vi "SV Continuous Swept-Sine THD+N.vi"(0 "scaled signals [EU]":waveform(dbl)[](array[waveform]), 1 "desired units":T3, 2 "reset? (F)":bool, 7 "harmonic range":cluster{"start order":dbl, "stop order":dbl}={"start order"=-1.0, "stop order"=-1.0} {"stop order" format="%.2f"; "start order" format="%.2f"}, 9 "advanced span [order]":dbl=1.0 format="%0.2f", 11 "error in (no error)":errorcluster, 12 "buffer settings":T2 {"buffer mode" items=["Infinite length", "Last block data", "Custom"]}, 13 "zero delay? (F)":bool) -> (3 "unit labels":T1(array[cluster]), 4 "scaled signals out [EU]":waveform(dbl)[](array[waveform]), 6 "THD+N":cluster{"frequency":dbl[], "amplitude":dbl[]}[](array[cluster]) {"amplitude" format="%.2f"; "frequency" format="%.2f"}, 8 "SINAD":cluster{"frequency":dbl[], "amplitude":dbl[]}[](array[cluster]) {"amplitude" format="%.2f"; "frequency" format="%.2f"}, 15 "error out":errorcluster)   [LabVIEW 2017, in "SoundVib_ContSweptSine.lvlib"]
doc: "Computes the total harmonic distortion plus noise (THD+N) and signal in noise and distortion (SINAD) of the input signals by performing a continuous swept-sine measurement."
uses:
  <vilib>/addons/Sound and Vibration/svt_Continuous Swept Sine/SoundVib_ContSweptSine.lvlib
  <vilib>/addons/_NISVFA/_Shared subVIs/Controls/sv_Buffer XY Settings.ctl
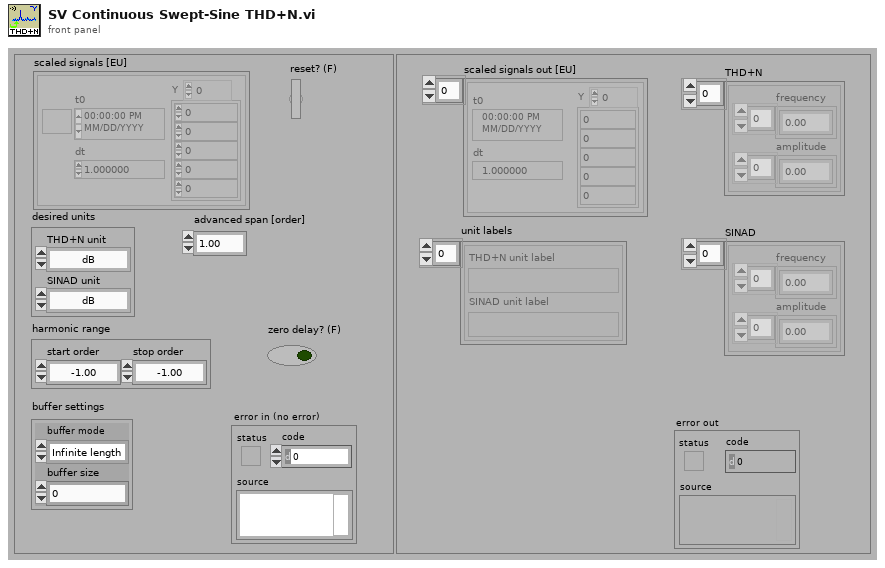
[diagram p1: front panel]
types:
  T1 = cluster{"THD+N unit label":string, "SINAD unit label":string}[]
  T2 = typedef "sv_Buffer XY Settings.ctl" = cluster{"buffer mode":u16, "buffer size":dbl}
  T3 = cluster{"THD+N unit":enum16{"dB", "linear ratio", "%"}, "SINAD unit":enum16{"dB", "linear ratio", "%"}}
  T4 = typedef "svc_Resampled Channel Info.ctl" = cluster{"channel name":string, "description":string, " channel info":T5}
  T5 = typedef "svc_Channel Info.ctl" = cluster{"sensor sensitivity":dbl, "engineering units":T6, "dB reference":dbl, "custom label":string, "weighting filter":T7, "pregain":dbl}
  T6 = typedef "svc_Engineering Units Text Ring.ctl" = u16
  T7 = typedef "svc_Weighting Filter Text Ring.ctl" = u16
  T8 = typedef "OAT Position Info.ctl" = cluster{"positions [s]":dbl[], "samples/rev":dbl}
  T9 = cluster{"THD+N unit":string, "SINAD unit":string}[]
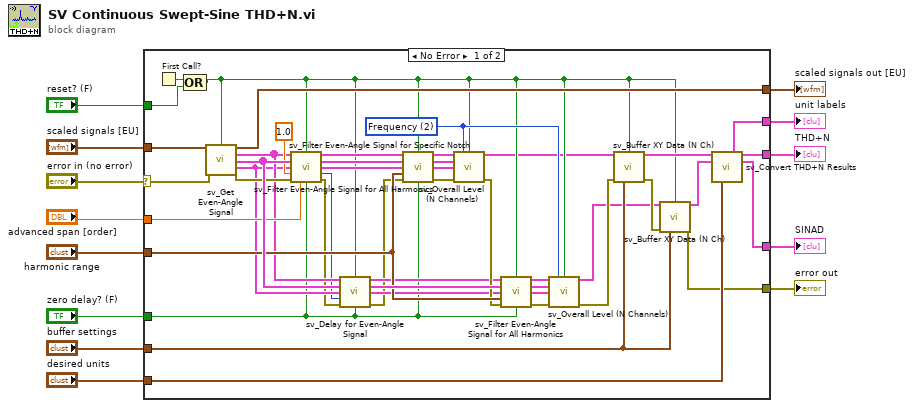
[diagram p0: block diagram]
diagram:
  n1 = case shown="No Error" "error in (no error)" {
    selector: "error in (no error)" -> [w54 w56]
    tunnel: [w35 w56] -> w12
    tunnel: "scaled signals [EU]" -> [w53 w55]
    tunnel: [w45 w55] -> w10
    tunnel: "desired units" -> [w36 _]
    tunnel: "harmonic range" -> [w29 _]
    tunnel: [w39 _] -> w7
    tunnel: [w38 _] -> w2
    tunnel: "buffer settings" -> [w44 _]
    tunnel: "zero delay? (F)" -> [w17 _]
    tunnel: "reset? (F)" -> [w46 _]
    tunnel: [w37 _] -> w3
    tunnel: "advanced span [order]" -> [w30 _]
    frame No Error {
      w50 = u16 2 items=["Time", "Revolution", "Frequency"] ("x-axis selection")
      n2 = First Call?() -> (First Call?: T/F=w47:bool)
      n3 = Compound Arithmetic op=OR(w47, w46) -> (w20:bool)
      n4 = call <vilib>:"sv_Get Even-Angle Signal.vi"("data to process"=w53, "reset?"=w20, "error in (no error)"=w54) -> ("data to process out"=w45:waveform(dbl)[], "even-angle signals"=w24:cluster{"r0":dbl, "dr":dbl, "Y":dbl[]}[], "even-angle channel info"=w52:T4[], "even-angle position info"=w22:T8, "error out"=w31:errorcluster)  [unwired: 7 in, 1 out]
      n5 = call <vilib>:"sv_Filter Even-Angle Signal for Specific Notch.vi"("even-angle signals"=w24, "reset?"=w20, "even-angle position info"=w22, "notch harmonic"=1.0, "error in (no error)"=w31, "bandwidth [order]"=w30, "zero delay? (F)"=w17) -> ("even-angle signals out"=w34:cluster{"r0":dbl, "dr":dbl, "Y":dbl[]}[], "even-angle position info out"=w33:T8, "delay [samples]"=w19:i32, "error out"=w18:errorcluster)  [unwired: 5 in]
      n6 = call <vilib>:"sv_Delay for Even-Angle Signal.vi"("even-angle signals"=w24, "reset?"=w20, "even-angle position info"=w22, "delay [samples]"=w19, "error in (no error)"=w18, "zero delay? (F)"=w17) -> ("even-angle signals out"=w23:cluster{"r0":dbl, "dr":dbl, "Y":dbl[]}[], "even-angle position info out"=w21:T8, "error out"=w16:errorcluster)  [unwired: 7 in]
      n7 = call <vilib>:"sv_Filter Even-Angle Signal for All Harmonics.vi"("even-angle signals"=w34, "reset?"=w20, "even-angle position info"=w33, "harmonic range"=w29, "error in (no error)"=w16, "zero delay? (F)"=w17) -> ("even-angle signals out"=w49:cluster{"r0":dbl, "dr":dbl, "Y":dbl[]}[], "even-angle position info out"=w48:T8, "error out"=w51:errorcluster)  [unwired: 7 in]
      n8 = call <vilib>:"sv_Overall Level (N Channels).vi"("even-angle signals"=w49, "x-axis selection"=w50, "reset? (F)"=w20, "even-angle channel info"=w52, "even-angle position info"=w48, "error in (no error)"=w51) -> ("overall levels"=w15:cluster{"time/rev/rpm":dbl[], "level":dbl[]}[], "error out"=w26:errorcluster)  [unwired: 6 in, 2 out]
      n9 = call <vilib>:"sv_Filter Even-Angle Signal for All Harmonics.vi"("even-angle signals"=w23, "reset?"=w20, "even-angle position info"=w21, "harmonic range"=w29, "error in (no error)"=w26, "zero delay? (F)"=w17) -> ("even-angle signals out"=w28:cluster{"r0":dbl, "dr":dbl, "Y":dbl[]}[], "even-angle position info out"=w27:T8, "error out"=w25:errorcluster)  [unwired: 7 in]
      n10 = call <vilib>:"sv_Overall Level (N Channels).vi"("even-angle signals"=w28, "x-axis selection"=w50, "reset? (F)"=w20, "even-angle channel info"=w52, "even-angle position info"=w27, "error in (no error)"=w25) -> ("overall levels"=w14:cluster{"time/rev/rpm":dbl[], "level":dbl[]}[], "error out"=w43:errorcluster)  [unwired: 6 in, 2 out]
      n11 = call <vilib>:"sv_Buffer XY Data (N Ch).vi"("XY signals"=w15, "reset? (F)"=w20, "error in (no error)"=w43, "buffer settings"=w44) -> ("buffered XY signals"=w41:cluster{"X":dbl[], "Y":dbl[]}[], "error out"=w42:errorcluster)  [unwired: 10 in]
      n12 = call <vilib>:"sv_Buffer XY Data (N Ch).vi"("XY signals"=w14, "reset? (F)"=w20, "error in (no error)"=w42, "buffer settings"=w44) -> ("buffered XY signals"=w40:cluster{"X":dbl[], "Y":dbl[]}[], "error out"=w35:errorcluster)  [unwired: 10 in]
      n13 = call <vilib>:"sv_Convert THD+N Results.vi"("Residue Magnitudes"=w41, "Total Magnitudes"=w40, "desired units"=w36) -> ("units"=w38:T9, "THD+N"=w39:cluster{"frequency":dbl[], "amplitude":dbl[]}[], "SINAD"=w37:cluster{"frequency":dbl[], "amplitude":dbl[]}[])  [unwired: 10 in]
    }
    frame Error {
    }
  }
  "error out" <- w12
  "THD+N" <- w7
  "scaled signals out [EU]" <- w10
  "SINAD" <- w3
  "unit labels" <- w2
